vi "Variancia_online.vi"(8 "error in (no error)":errorcluster, 10 "M":dbl, 11 "u":dbl) -> (0 "error out":errorcluster, 1 "std":dbl, 2 "var":dbl, 3 "y":dbl)   [LabVIEW 2020]
panel:
  in  "Tab Control":enum32{"Page 1", "Page 2"}(tab)
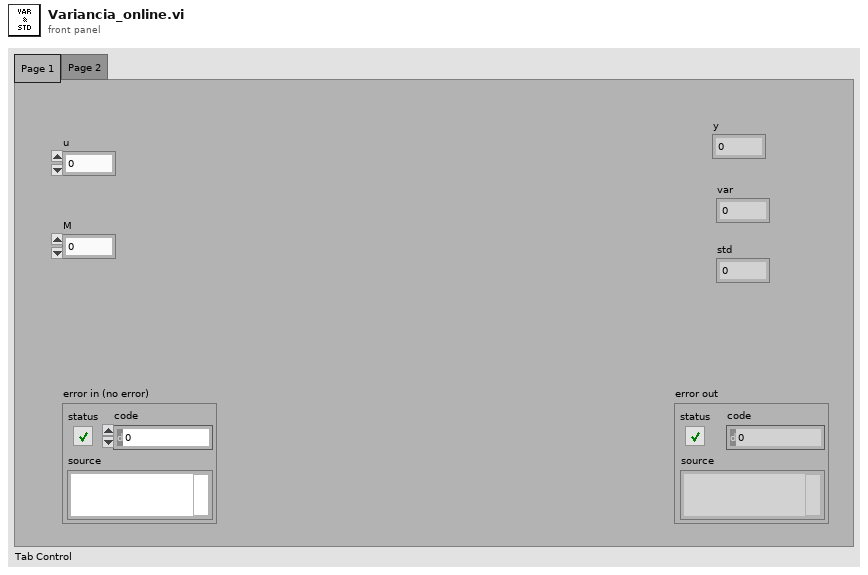
[diagram p1: front panel]
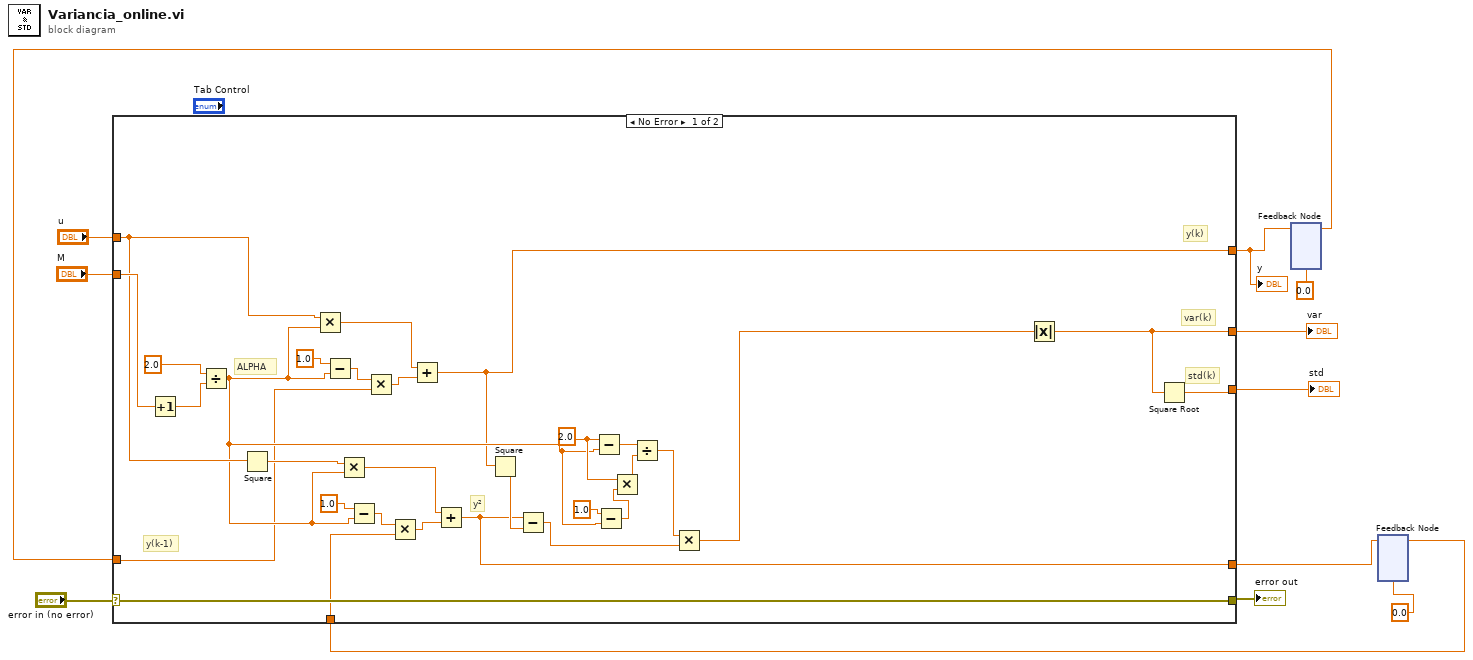
[diagram p0: block diagram]
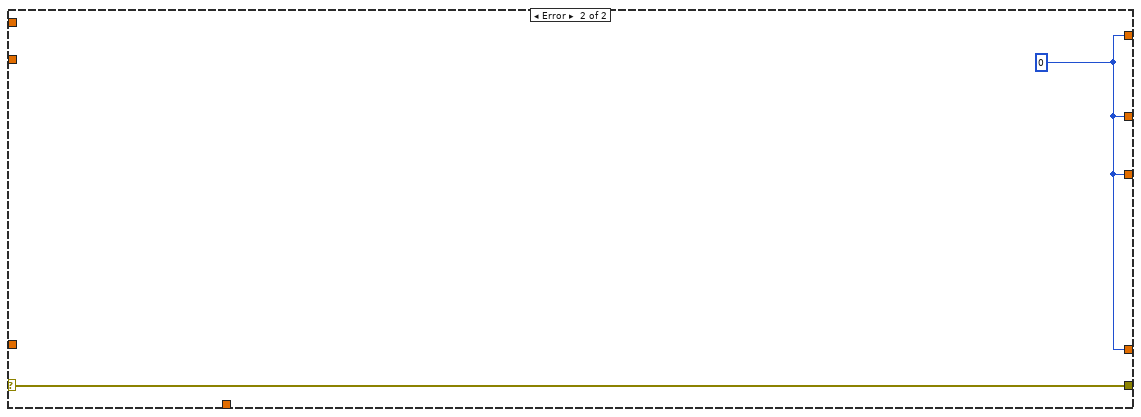
[diagram p2: hidden frame]
diagram:
  n1 = feedback #1(0.0) -> (w6:dbl)
  n2 = feedback #2(0.0) -> (w1:dbl)
  n3 = case shown="No Error" "error in (no error)" {
    selector: "error in (no error)" -> [w42 w44]
    tunnel: "M" -> [w39 _]
    tunnel: "u" -> [w30 _]
    tunnel: [w42 w44] -> w9
    tunnel: [w22 w43] -> w4
    tunnel: [w13 w43] -> w8
    tunnel: [w18 w43] -> w7
    tunnel: w6 -> [w17 _]
    tunnel: [w16 w43] -> w2
    tunnel: w1 -> [w15 _]
    frame No Error {
      w27 = 2.0
      # "std(k)"
      # "var(k)"
      # "y(k)"
      # "y(k-1)"
      # "y²"
      # "ALPHA"
      n4 = Increment(x=w39) -> (x+1=w40:dbl)
      n5 = Divide(x=2.0, y=w40) -> (x/y=w25:dbl)
      n6 = Square(x=w30) -> (x^2=w29:dbl)
      n7 = Multiply(x=w30, y=w25) -> (x*y=w35:dbl)
      n8 = Subtract(x=1.0, y=w25) -> (x-y=w38:dbl)
      n9 = Multiply(x=w29, y=w25) -> (x*y=w34:dbl)
      n10 = Subtract(x=1.0, y=w25) -> (x-y=w31:dbl)
      n11 = Multiply(x=w38, y=w17) -> (x*y=w37:dbl)
      n12 = Multiply(x=w31, y=w15) -> (x*y=w32:dbl)
      n13 = Add(x=w35, y=w37) -> (x+y=w22:dbl)
      n14 = Add(x=w34, y=w32) -> (x+y=w16:dbl)
      n15 = Square(x=w22) -> (x^2=w21:dbl)
      n16 = Subtract(x=w16, y=w21) -> (x-y=w20:dbl)
      n17 = Subtract(x=w27, y=w25) -> (x-y=w28:dbl)
      n18 = Subtract(x=1.0, y=w25) -> (x-y=w24:dbl)
      n19 = Multiply(x=w27, y=w24) -> (x*y=w23:dbl)
      n20 = Divide(x=w28, y=w23) -> (x/y=w19:dbl)
      n21 = Multiply(x=w19, y=w20) -> (x*y=w14:dbl)
      n22 = Absolute Value(x=w14) -> (abs(x)=w13:dbl)
      n23 = Square Root(x=w13) -> (sqrt(x)=w18:dbl)
    }
    frame Error {
      w43 = 0
    }
  }
  "y" <- w4
  "error out" <- w9
  "std" <- w7
  "var" <- w8
  n24 = feedback-in #1(w4) -> ()
  n25 = feedback-in #2(w2) -> ()
